vi "Timer_Cycle_Code.vi"(9 "Burner OFF Time (Seconds)":dbl, 10 "Burner ON Time (Seconds)":dbl, 11 "Timer":dbl) -> (3 "burner_state":dbl)   [LabVIEW 2023]
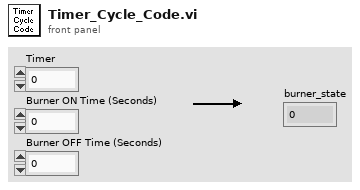
[diagram p1: front panel]
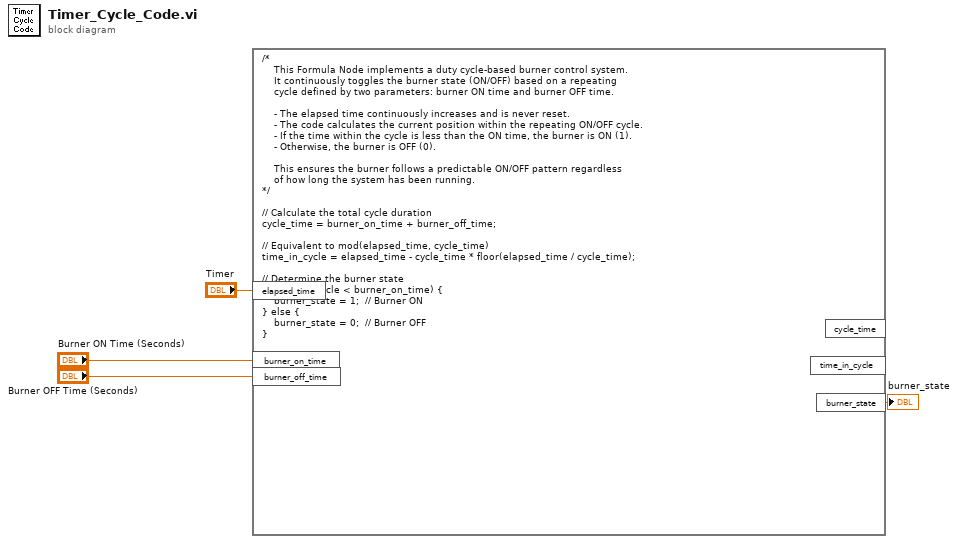
[diagram p0: block diagram]
diagram:
  n1 = formula code="/*\n    This Formula Node implements a duty cycle-based burner control system. \n    It continuously toggles the burner state (ON/OFF) based on a repeating \n    cycle defined by two parameters: burner ON time and burner OFF time. \n\n    - The elapsed time continuously increases and is never reset.\n    - The code calculates the current position within the repeating ON/OFF cycle.\n    - If the time within the cycle is less than the ON time, the burner is ON (1).\n    - Otherwise, the burner is OFF (0).\n\n    This ensures the burner follows a predictable ON/OFF pattern regardless \n    of how long the system has been running.\n*/\n\n// Calculate the total cycle duration\ncycle_time = burner_on_time + burner_off_time;\n\n// Equivalent to mod(elapsed_time, cycle_time)\ntime_in_cycle = elapsed_time - cycle_time * floor(elapsed_time / cycle_time);\n\n// Determine the burner state\nif (time_in_cycle < burner_on_time) {\n    burner_state = 1;  // Burner ON\n} else {\n    burner_state = 0;  // Burner OFF\n}"("burner_on_time"="Burner ON Time (Seconds)", "burner_off_time"="Burner OFF Time (Seconds)", "elapsed_time"="Timer") -> ("burner_state"=→"burner_state":dbl)  [unwired: 2 out]
